vi "Convert 1D to 2D.vi"   [LabVIEW 2014]
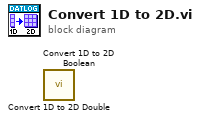
[diagram p0: block diagram]
diagram:
  n1 = call "Convert 1D to 2D Double.vi"() -> ()  [unwired: 11 in, 1 out]
  n2 = call "Convert 1D to 2D Boolean.vi"() -> ()  [unwired: 11 in, 1 out]
